vi "Unubscribe Request.vi"(8 "error in (no error)":errorcluster, 9 "Subscriber":string, 10 "Topic":string, 11 "Measure Object in":refnum<class "Measure Object.lvclass">) -> (0 "error out":errorcluster, 3 "Measure Object out":refnum<class "Measure Object.lvclass">)   [LabVIEW 2015, in "Measure Object.lvclass"]
uses:
  Measure Object.lvclass
  Measure Object.lvclass/Measure Object.ctl
  BroadcastBroker/BroadcastBroker.lvclass
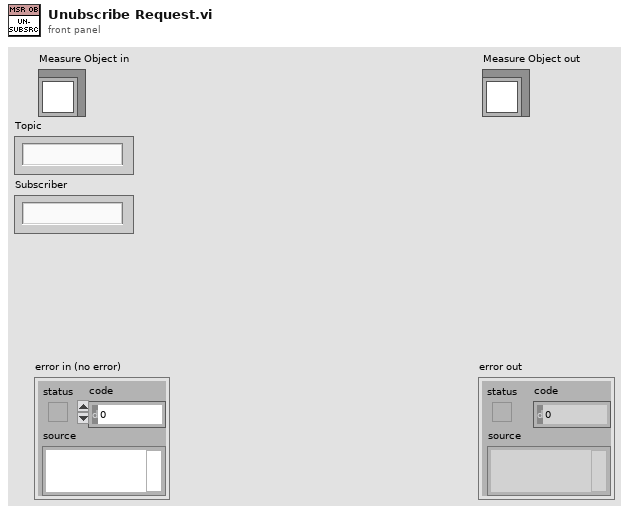
[diagram p1: front panel]
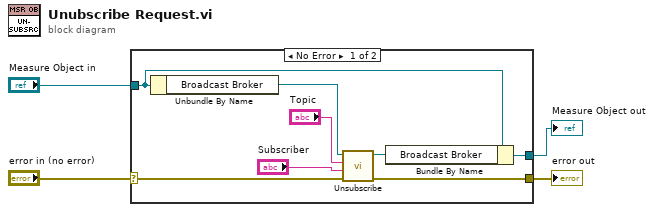
[diagram p0: block diagram]
diagram:
  n1 = case shown="No Error" "error in (no error)" {
    selector: "error in (no error)" -> [w8 w14]
    tunnel: [w7 w14] -> w3
    tunnel: [w6 w13] -> w1
    tunnel: "Measure Object in" -> [w12 w13]
    frame No Error {
      n2 = Unbundle By Name(w12) -> ("Broadcast Broker"=w11:refnum<class "BroadcastBroker.lvclass">)
      n3 = call-dynamic "Unsubscribe.vi"("error in (no error)"=w8, "Subscriber"="Subscriber", "Topic"="Topic", "Broadcaster in"=w11) -> ("error out"=w7:errorcluster, "Broadcaster out"=w5:refnum<class "BroadcastBroker.lvclass">)  [unwired: 6 in]
      n4 = Bundle By Name(cluster=w12, "Broadcast Broker"=w5) -> (w6:refnum<class "Measure Object.lvclass">)
    }
    frame Error {
    }
  }
  "error out" <- w3
  "Measure Object out" <- w1
